vi "Score Particle.vi"(11 "Particle Values":dbl[](array[numeric])) -> (0 "Rect":T1, 3 "Scores":T2)   [LabVIEW 2019]
panel:
  # "This code assumes that the\nparticle measurements are ...\n0. The particle area\n1. Bounding box left\n2. Bounding box top\n3. Bounding box right\n4. Bounding box bottom\n5. Orientation\n6. Type Factor\n7. Normalized MoI XX\n8. Normalized MoI yy\n9. Holes' Area\n10. Convex Hull Area\n\nIt calculates the output scores\nfor each particle."
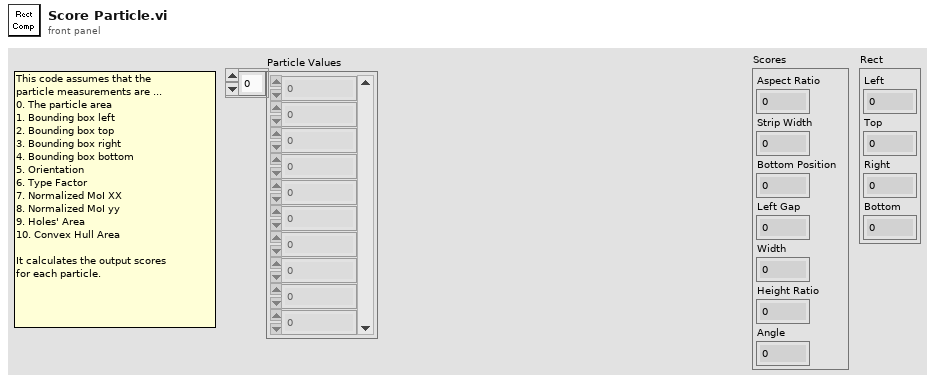
[diagram p1: front panel]
types:
  T1 = cluster{"Left":dbl, "Top":dbl, "Right":dbl, "Bottom":dbl}
  T2 = cluster{"Aspect Ratio":dbl, "Strip Width":dbl, "Bottom Position":dbl, "Left Gap":dbl, "Width":dbl, "Height Ratio":dbl, "Angle":dbl}
  T3 = cluster{"[0]":dbl, "[1]":dbl, "[2]":dbl, "[3]":dbl}
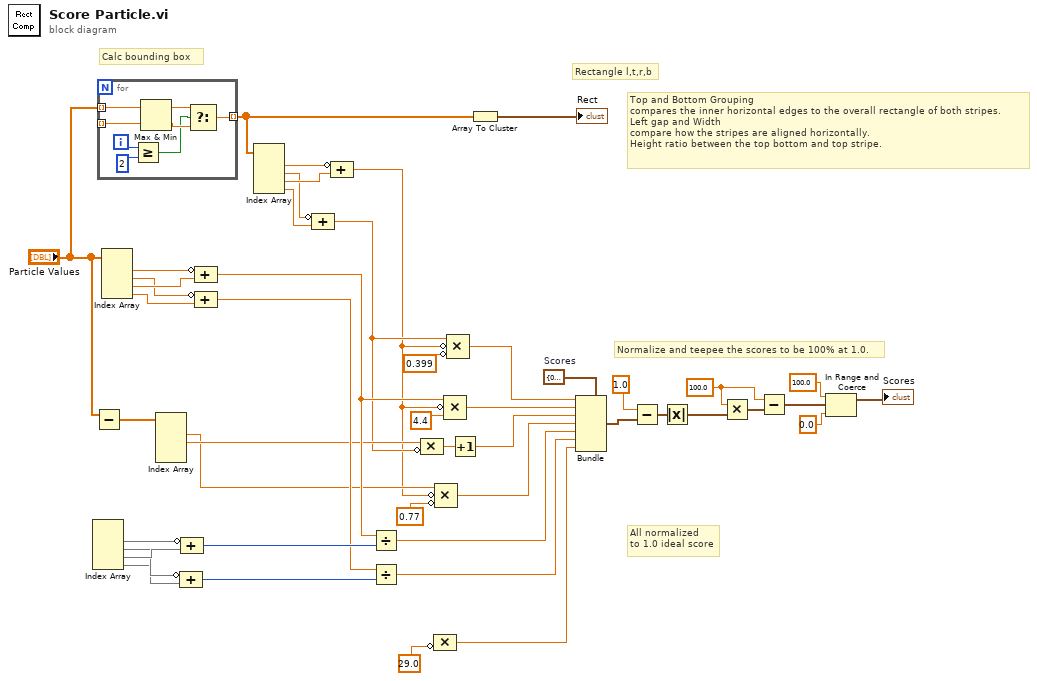
[diagram p0: block diagram]
diagram:
  w1 = T2 {"Aspect Ratio"=0.0, "Strip Width"=0.0, "Bottom Position"=0.0, "Left Gap"=0.0, "Width"=0.0, "Height Ratio"=0.0, "Angle"=0.0}  # Scores
  w35 = 100.0 ("x/y")
  # "All normalized\nto 1.0 ideal score"
  # "Normalize and teepee the scores to be 100% at 1.0."
  # "Top and Bottom Grouping\ncompares the inner horizontal edges to the overall rectangle of both stripes.\nLeft gap and Width\ncompare how the stripes are aligned horizontally.\nHeight ratio between the top bottom and top stripe."
  # "Calc bounding box"
  # "Rectangle l,t,r,b"
  n1 = Index Array() -> (element #1=w45, element #2=w26, element #3=w48, element #4=w11)  [unwired: 5 in]
  n2 = Subtract(x="Particle Values") -> (x-y=w17:dbl[])  [unwired: 1 in]
  n3 = for {
    tunnel: "Particle Values" -> [w56] mode=indexing
    tunnel: _ -> [w55] mode=indexing
    tunnel: [w49] -> w20 mode=indexing
    i -> [w53]
    n4 = Greater Or Equal?(x=w53, y=2) -> (x >= y?=w50:bool)
    n5 = Max & Min(x=w56, y=w55) -> (max(x,y)=w52:dbl, min(x,y)=w51:dbl)
    n6 = Select(t=w52, s=w50, f=w51) -> (s? t:f=w49:dbl)
  }
  n7 = Index Array(array="Particle Values") -> (element #1=w40:dbl, element #2=w25:dbl, element #3=w39:dbl, element #4=w41:dbl)  [unwired: 4 in]
  n8 = Index Array(array=w17) -> (element #1=w15:dbl, element #2=w16:dbl)  [unwired: 4 in, 2 out]
  n9 = Compound Arithmetic op=ADD(invert w26, w11) -> (w46:i32)
  n10 = Compound Arithmetic op=ADD(invert w45, w48) -> (w47:i32)
  n11 = Compound Arithmetic op=ADD(invert w40, w39) -> (w23:dbl)
  n12 = Compound Arithmetic op=ADD(invert w25, w41) -> (w27:dbl)
  n13 = Index Array(array=w20) -> (element #1=w13:dbl, element #2=w10:dbl, element #3=w12:dbl, element #4=w9:dbl)  [unwired: 4 in]
  n14 = Compound Arithmetic op=ADD(invert w10, w9) -> (w8:dbl)
  n15 = Compound Arithmetic op=ADD(invert w13, w12) -> (w7:dbl)
  n16 = Divide(x=w23, y=w47) -> (x/y=w43:dbl)
  n17 = Divide(x=w27, y=w46) -> (x/y=w42:dbl)
  n18 = Compound Arithmetic op=MULTIPLY(w16, invert w8) -> (w22:dbl)
  n19 = Compound Arithmetic op=MULTIPLY(invert 29.0 ("y")) -> (w2:dbl, w4:dbl)
  n20 = Compound Arithmetic op=MULTIPLY(w15, invert w7, invert 0.77 ("y")) -> (w18:dbl)
  n21 = Compound Arithmetic op=MULTIPLY(w23, invert w7, 4.4 ("y")) -> (w44:dbl)
  n22 = Compound Arithmetic op=MULTIPLY(w8, invert w7, invert 0.399 ("y")) -> (w5:dbl)
  n23 = Increment(x=w22) -> (x+1=w21:dbl)
  n24 = Array To Cluster(array=w20) -> (cluster=→"Rect":T3)
  n25 = Bundle(cluster=w1, "Aspect Ratio"=w5, "Strip Width"=w44, "Bottom Position"=w21, "Left Gap"=w18, "Width"=w43, "Height Ratio"=w42, "Angle"=w2) -> (w29:T2)
  n26 = Subtract(x=1.0 ("y"), y=w29) -> (x-y=w33:T2)
  n27 = Absolute Value(x=w33) -> (abs(x)=w36:T2)
  n28 = Multiply(x=w35, y=w36) -> (x*y=w37:T2)
  n29 = Subtract(x=w35, y=w37) -> (x-y=w32:T2)
  n30 = In Range and Coerce(upper limit=100.0, x=w32, lower limit=0.0) -> (coerced(x)=→"Scores":T2)  [unwired: 1 out]
